vi "Set OPC Timeout.vi"(8 "error in (no error)":errorcluster, 10 "OPC Timeout":i32=30000, 11 "VISA resource name":refnum<visa-resource-name>) -> (0 "error out":errorcluster, 3 "VISA resource name out":refnum<visa-resource-name>)   [LabVIEW 2020, in "Rohde&Schwarz CMXP GPRF.lvlib"]
doc: "This VI sets the value of the driver's OPC timeout in milliseconds. OPC timeout is different from the VISA timeout and it is used by the instrument driver for long-lasting operations, e.g. instrument's acquisition."
uses:
  <instrlib>/Rohde&Schwarz CMXP GPRF/Rohde&Schwarz CMXP GPRF.lvlib
  <instrlib>/Rohde&Schwarz CMXP GPRF/Private/rsidr_core.llb/type_Session_Parameter_int32.ctl
  <instrlib>/Rohde&Schwarz CMXP GPRF/Private/rsidr_core.llb/rsidr_core.lvlib
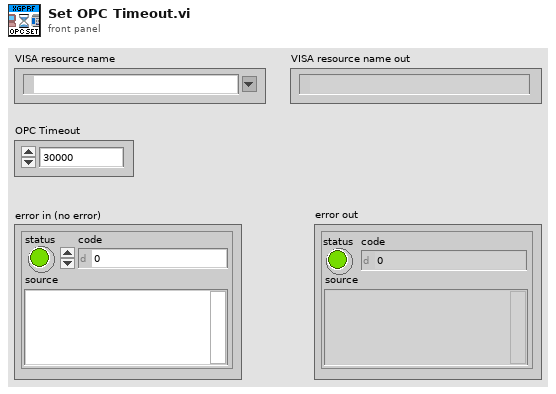
[diagram p1: front panel]
types:
  T1 = typedef "Rohde&Schwarz CMXP GPRF.lvlib/rsidr_core.lvlib/type_Session_Parameter_int32.ctl" = enum16{"OPC Timeout", "Additional Flags", "Wait Before Write", "Wait Before Read", "Bin Data Chunk Size", "VISA Access Mode", "VISA Timeout", "Bin Float Number Format", "Bin Integer Number Format", "STBpollVISAtimeout", "OPCwaitMode"}
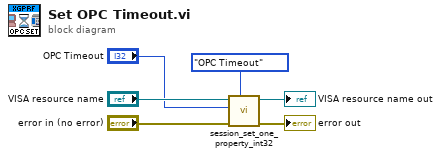
[diagram p0: block diagram]
diagram:
  n1 = call <instrlib>:"session_set_one_property_int32.vi"("Session Parameter Integer"=type_Session_Parameter_int32."OPC Timeout" ("Session Parameter to set"), "error in"="error in (no error)", "Int32 value in"="OPC Timeout", "VISA resource name"="VISA resource name") -> ("error out"=→"error out":errorcluster, "VISA resource name out"=→"VISA resource name out":refnum<visa-resource-name>)  [unwired: 5 in, 1 out]
